vi "ProgramControlStateTracker.vi"(0 "Universal Robot.lvclass":refnum<class "Universal Robot.lvclass">, 5 "Complete (F)":bool, 6 "State in":string, 8 "Program":string) -> (14 "Universal Robot.lvclass out":refnum<class "Universal Robot.lvclass">)   [LabVIEW 2019, in "Universal Robot.lvclass"]
uses:
  Universal Robot.lvclass
  Universal Robot.lvclass/Universal Robot.ctl
  <vilib>/Utility/file.llb/Write Delimited Spreadsheet (string).vi
panel:
  out "States":string[][](array[string])
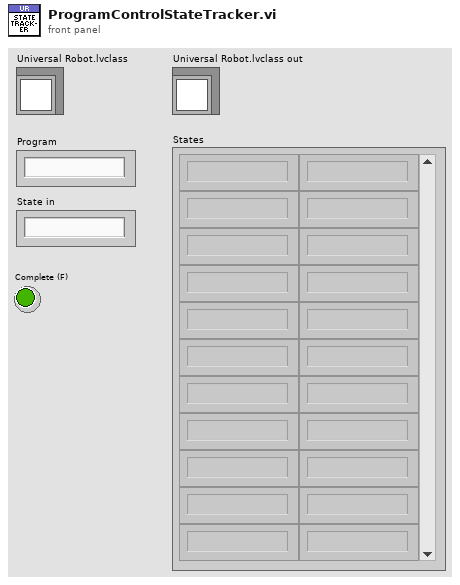
[diagram p1: front panel]
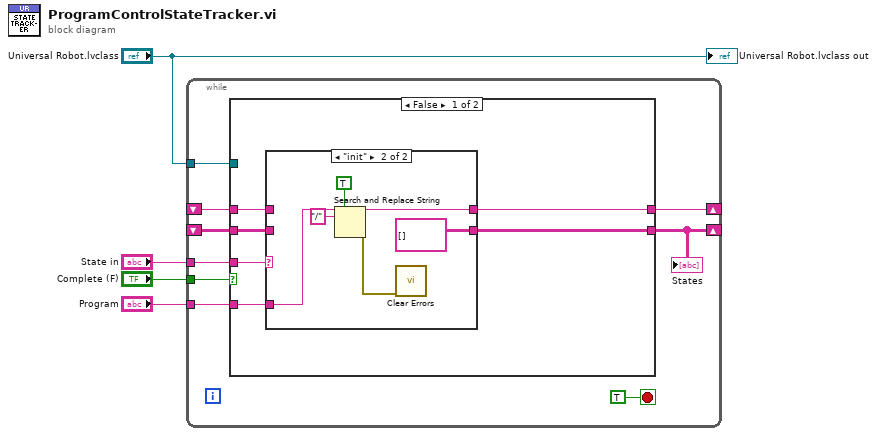
[diagram p0: block diagram]
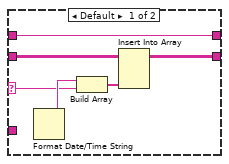
[diagram p2: hidden frame]
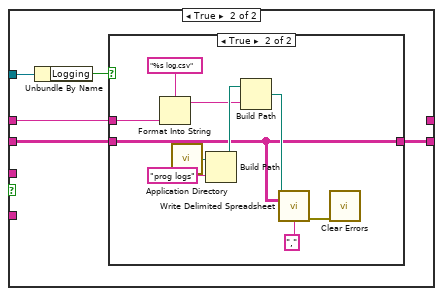
[diagram p3: hidden frame]
diagram:
  n1 = while {
    tunnel: "State in" -> [w9]
    shift-right: [w12] -> _
    shift-left: _ -> [w11]
    tunnel: "Complete (F)" -> [w10]
    shift-right: [w6] -> _
    shift-left: _ -> [w8]
    tunnel: "Program" -> [w7]
    tunnel: "Universal Robot.lvclass" -> [w5]
    stop <- TRUE stop-if-true
    n2 = case shown="False" w10 {
      tunnel: [w19 w34] -> w12
      tunnel: w11 -> [w18 w35]
      tunnel: w9 -> [w17 _]
      tunnel: w8 -> [w14 w36]
      tunnel: w7 -> [w16 _]
      tunnel: [w15 _] -> w6
      tunnel: w5 -> [_ w33]
      frame False {
        n3 = case shown="\"init\"" w17 {
          selector: w17 -> [w20 _]
          tunnel: [w25 string[][] []] -> w19
          tunnel: w18 -> [w24 _]
          tunnel: w16 -> [_ w30]
          tunnel: [w22 w29] -> w15
          tunnel: w14 -> [w22 _]
          frame Default {
            n4 = Format Date/Time String() -> (date/time string=w21:string)  [unwired: 3 in]
            n5 = Build Array(w21, w20) -> (w23:string[])
            n6 = Insert Into Array(array=w24, new element=w23) -> (w25:string[][])  [unwired: 2 in]
          }
          frame "init" {
            n7 = Search and Replace String(replace all?=TRUE ("replace all? (F)"), input string=w30, search string="/") -> (result string=w29:string, error out=w26:errorcluster)  [unwired: 5 in, 2 out]
            n8 = call <vilib>:"Clear Errors.vi"("error in (no error)"=w26) -> ()  [unwired: 5 in, 2 out]
          }
        }
      }
      frame True {
        n9 = Unbundle By Name(w33) -> ("Logging"=w32:bool)
        n10 = case shown="True" w32 {
          tunnel: w36 -> [_ w47]
          tunnel: w35 -> [w37 w38]
          tunnel: [w37 w38] -> w34
          frame False {
          }
          frame True {
            n11 = Format Into String(format string="%s log.csv", w47) -> (resulting string=w39:string)  [unwired: 2 in, 1 out]
            n12 = call <vilib>:"Application Directory.vi"() -> ("Application Directory"=w45:path)
            n13 = Build Path(base path=w45, name or relative path="prog logs") -> (appended path=w41:path)
            n14 = Build Path(base path=w41, name or relative path=w39) -> (appended path=w40:path)
            n15 = call-poly <vilib>:"Write Delimited Spreadsheet.vi"("file path (dialog if empty)"=w40, "2D data"=w38, "delimiter (\\t)"="," ("delimiter (\\t)")) -> ("error out"=w44:errorcluster)  [unwired: 11 in, 1 out]
            n16 = call <vilib>:"Clear Errors.vi"("error in (no error)"=w44) -> ()  [unwired: 5 in, 2 out]
          }
        }
      }
    }
    "States" <- w12
  }
  "Universal Robot.lvclass out" <- "Universal Robot.lvclass"
